vi "Write Header.vi"(8 "error in":errorcluster, 10 "Header":string[](array[string]), 11 "SLL in":refnum<class "SLL.lvclass">) -> (0 "error out":errorcluster, 3 "SLL out":refnum<class "SLL.lvclass">)   [LabVIEW 2023, in "SLL.lvlib" / "SLL.lvclass"]
uses:
  SLL.lvclass
  SLL.lvclass/SLL.ctl
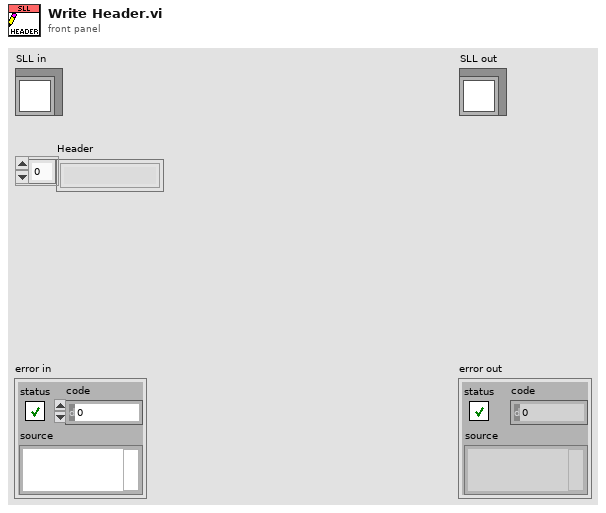
[diagram p1: front panel]
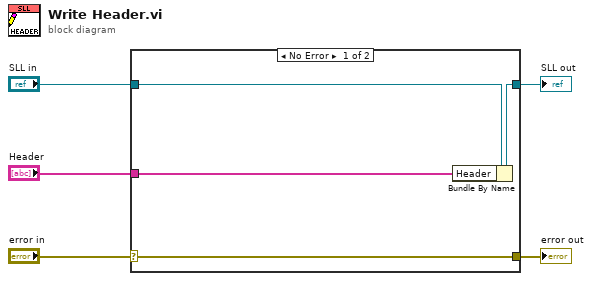
[diagram p0: block diagram]
diagram:
  n1 = case shown="No Error" "error in" {
    selector: "error in" -> [w9 w10]
    tunnel: [w9 w10] -> w4
    tunnel: [w7 w11] -> w2
    tunnel: "SLL in" -> [w8 w11]
    tunnel: "Header" -> [w6 _]
    frame No Error {
      n2 = Bundle By Name(cluster=w8, "Header"=w6) -> (w7:refnum<class "SLL.lvclass">)
    }
    frame Error {
    }
  }
  "error out" <- w4
  "SLL out" <- w2
